vi "sync Write Tx Only.vi"(6 "param_length":u16, 7 "data_length":u16, 9 "start_address":u16, 10 "protocol_version":i32, 11 "port_num":i32) -> ()   [LabVIEW 2016, in "dxl_x86_c.lvlib"]
doc: "WINDECLSPEC void syncWriteTxOnly (int port_num, int protocol_version, uint16_t start_address, uint16_t data_length, uint16_t param_length);"
uses:
  dxl_x86_c.lvlib
  dxl_x86_c.dll
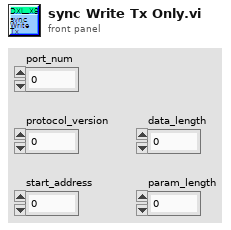
[diagram p1: front panel]
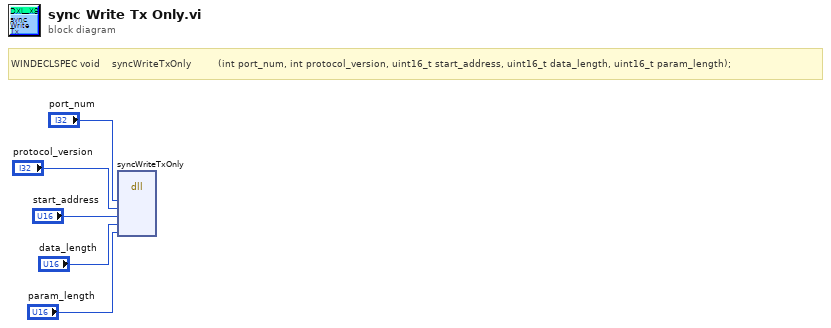
[diagram p0: block diagram]
diagram:
  # "WINDECLSPEC void    syncWriteTxOnly         (int port_num, int protocol_version, uint16_t start_address, uint16_t data_length, uint16_t param_length);"
  n1 = dll-call lib="C:/Users/Platform/Desktop/DynamixelSDK/labview/dxl_x86_c.lvlib/dxl_x86_c.*" fn="syncWriteTxOnly"("port_num"="port_num", "protocol_version"="protocol_version", "start_address"="start_address", "data_length"="data_length", "param_length"="param_length") -> ()  [unwired: 9 in, 2 out]
